vi "Draw Circle(SubVI).vi"(9 "Circle Index":i32, 11 "Circles":T2(array[cluster])) -> (0 "element":T1, 2 "Score":dbl, 3 "Bounding Rectangle out":T3)   [LabVIEW 2014]
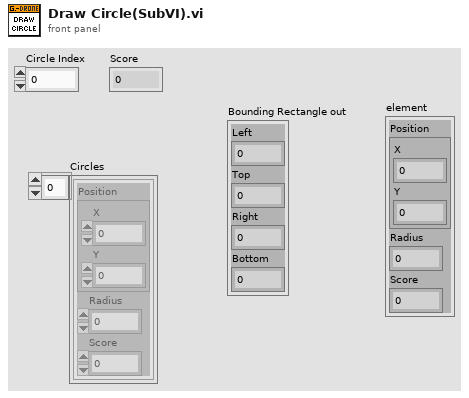
[diagram p1: front panel]
types:
  T1 = cluster{"Position":cluster{"X":sgl, "Y":sgl}, "Radius":dbl, "Score":dbl}
  T2 = cluster{"Position":cluster{"X":sgl, "Y":sgl}, "Radius":dbl, "Score":dbl}[]
  T3 = cluster{"Left":i32, "Top":i32, "Right":i32, "Bottom":i32}
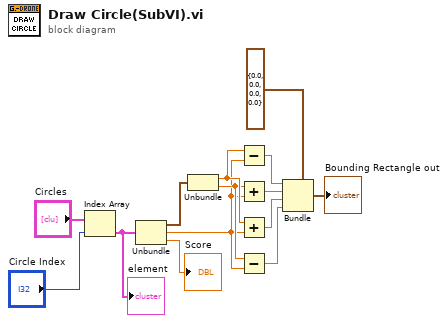
[diagram p0: block diagram]
diagram:
  n1 = Index Array(array="Circles", index="Circle Index") -> (element=w2:T1)
  "element" <- w2
  n2 = Unbundle(w2) -> ("Position"=w13:cluster{"X":sgl, "Y":sgl}, "Radius"=w9:dbl, "Score"=→"Score":dbl)
  n3 = Unbundle(w13) -> ("X"=w11:sgl, "Y"=w10:sgl)
  n4 = Subtract(x=w11, y=w9) -> (x-y=w8:dbl)
  n5 = Add(x=w10, y=w9) -> (x+y=w7:dbl)
  n6 = Add(x=w11, y=w9) -> (x+y=w6:dbl)
  n7 = Subtract(x=w10, y=w9) -> (x-y=w5:dbl)
  n8 = Bundle(cluster=cluster{dbl, dbl, dbl, dbl} {0.0, 0.0, 0.0, 0.0}, w8, w7, w6, w5) -> (→"Bounding Rectangle out":cluster{dbl, dbl, dbl, dbl})
